vi "Byte_read.vi"(2 "DUT":i32, 3 "Bit index":i32, 4 "index":i32=1) -> (0 "element":bool, 1 "0, 1":i16)   [LabVIEW 2024, in "Test_2.lvlib"]
uses:
  Test_2.lvlib
  PCANusb_DTU/support/PCAN_Global.vi
  PCANusb_DTU/PCANusb_DTU.lvlib
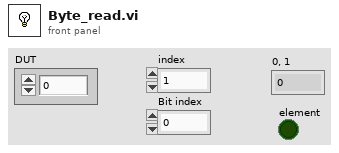
[diagram p1: front panel]
types:
  T1 = typedef "XNET Frame CAN.ctl" = cluster{"timestamp":timestamp, "payload":u8[], "identifier":u32, "type":T2, "extended?":bool, "echo?":bool}
  T2 = typedef "XNET Frame Type CAN.ctl" = u8
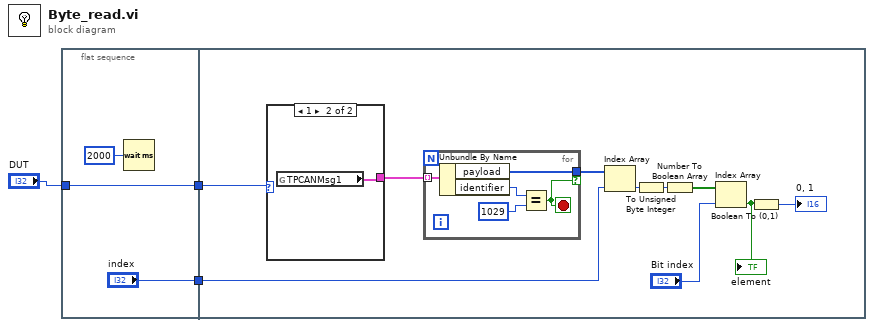
[diagram p0: block diagram]
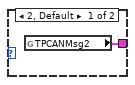
[diagram p2: hidden frame]
diagram:
  n1 = flat-sequence {
    tunnel: [w6] -> w3
    tunnel: "DUT" -> [w6]
    tunnel: ["index"] -> w1
    tunnel: w3 -> [w8]
    tunnel: w1 -> [w7]
    frame #0 {
      n2 = Wait (ms)(milliseconds to wait=u32 2000) -> ()  [unwired: 1 out]
    }
    frame #1 {
      n3 = case shown="1" w8 {
        tunnel: [w22 w23] -> w13
        frame 2, Default {
          n4 = global read "PCAN_Global.vi" "TPCANMsg2"() -> (w22:T1[])
        }
        frame 1 {
          n5 = global read "PCAN_Global.vi" "TPCANMsg1"() -> (w23:T1[])
        }
      }
      n6 = for {
        tunnel: [w19] -> w16 if=w18
        tunnel: w13 -> [w17] mode=indexing
        stop <- w18 stop-if-true
        n7 = Unbundle By Name(w17) -> ("payload"=w19:u8[], "identifier"=w20:u32)
        n8 = Equal?(x=w20, y=u32 1029 ("identifier")) -> (x = y?=w18:bool)
      }
      n9 = Index Array(array=w16, index=w7) -> (element=w15:u8)
      n10 = To Unsigned Byte Integer(number=w15) -> (unsigned 8bit integer=w14:u8)
      n11 = Number To Boolean Array(number=w14) -> (Boolean array=w12:bool[])
      n12 = Index Array(array=w12, index="Bit index") -> (element=w11:bool)
      "element" <- w11
      n13 = Boolean To (0,1)(Boolean=w11) -> (0, 1=→"0, 1":i16)
    }
  }
